vi "Create APP UI Display Events.vi"(11 "error in":errorcluster) -> (4 "UI.Event References":T1, 15 "error out":errorcluster)   [LabVIEW 2026, in "Synchronize AWS S3 Content.lvlib"]
doc: "Create resources for UI user events.\n\n<B>Input Parameters</B>\n\n<B>error in</B> describes error conditions that occur before this node runs. This input provides standard error in functionality.\n\n<B>Output Parameters</B>\n\n<B>UI display events out</B> created user events.\n\n<B>error out</B> contains error information. This output provides standard error out functionality."
uses:
  Synchronize AWS S3 Content.lvlib
  Core Components/Dependencies/TLB`_Dependencies.lvlib
  _UI APP Event References.ctl
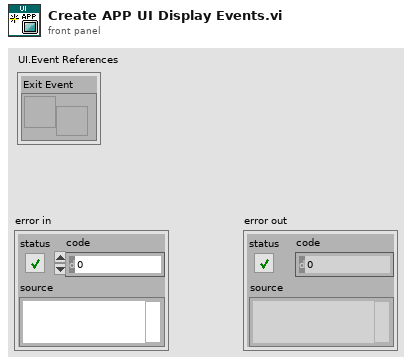
[diagram p1: front panel]
types:
  T1 = typedef "Synchronize AWS S3 Content.lvlib/_UI APP Event References.ctl" = cluster{"Exit Event":refnum<user-event>}
  T2 = typedef "Synchronize AWS S3 Content.lvlib/TLB`_Dependencies.lvlib/Exit Event Ref.ctl" = refnum<user-event>
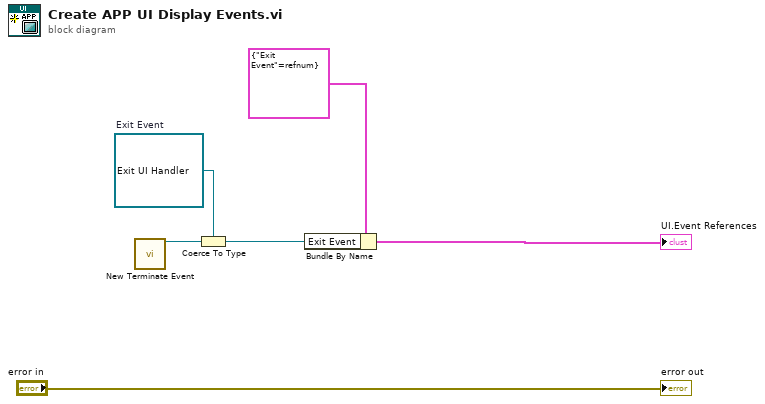
[diagram p0: block diagram]
diagram:
  w3 = refnum<user-event> refnum  # Exit Event
  n1 = call "New Terminate Event.vi"() -> ("Exit Event Ref"=w6:T2)  [unwired: 14 in, 1 out]
  n2 = Coerce To Type(0:w6, 1:w3) -> (2:w5:refnum<user-event>)
  n3 = Bundle By Name(cluster=T1 {"Exit Event"=refnum} ("UI.Event References 2"), "Exit Event"=w5) -> (→"UI.Event References":T1)
  "error out" <- "error in"
